vi "16- Random number in a text file.vi"() -> ()   [LabVIEW 2019]
panel:
  in  "Give file path to write data":path
  in  "?":bool
  # "Write random number in the range of 0 to 10 in the given text file"
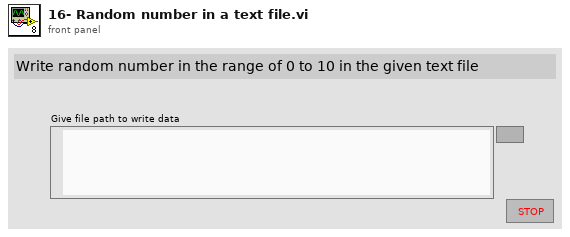
[diagram p1: front panel]
types:
  T1 = enum16{"open", "replace", "create", "open or create", "replace or create", "replace or create with confirmation"}
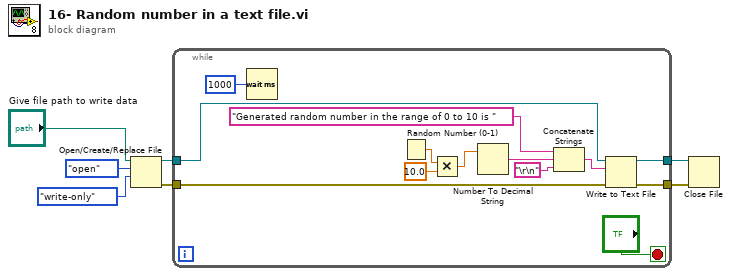
[diagram p0: block diagram]
diagram:
  n1 = Open/Create/Replace File(file path (use dialog)="Give file path to write data", operation (0:open)=T1."open", access (0:read/write)=enum16{"read/write", "read-only", "write-only"}."write-only") -> (refnum out=w2:refnum<file>, error out=w7:errorcluster)  [unwired: 3 in, 1 out]
  n2 = while {
    tunnel: w7 -> [w19]
    tunnel: [w18] -> w6
    tunnel: w2 -> [w17]
    tunnel: [w16] -> w1
    stop <- "?" stop-if-true
    n3 = Wait (ms)(milliseconds to wait=u32 1000) -> ()  [unwired: 1 out]
    n4 = Random Number (0-1)() -> (number: 0 to 1=w15:dbl)
    n5 = Multiply(x=w15, y=10.0) -> (x*y=w13:dbl)
    n6 = Number To Decimal String(number=w13) -> (decimal integer string=w12:string)  [unwired: 1 in]
    n7 = Concatenate Strings("Generated random number in the range of 0 to 10 is " ("string"), w12, "\r\n") -> (w9:string)
    n8 = Write to Text File(file (use dialog)=w17, text=w9, error in=w19) -> (refnum out=w16:refnum<file>, error out=w18:errorcluster)  [unwired: 1 in, 1 out]
  }
  n9 = Close File(refnum=w1, error in=w6) -> ()  [unwired: 2 out]
